vi "Variant_AdaptToType.vi"(7 "Default Type":variant, 10 "Variant":variant, 11 "Name (Default Type name)":string) -> (2 "Adapted Variant":variant)   [LabVIEW 2013, in "OpenVariant.lvlib"]
uses:
  OpenVariant.lvlib
  TypeDescriptor/TypeDescriptor_GetName.vi
  TypeDescriptor/TypeDescriptor_GetPString.vi
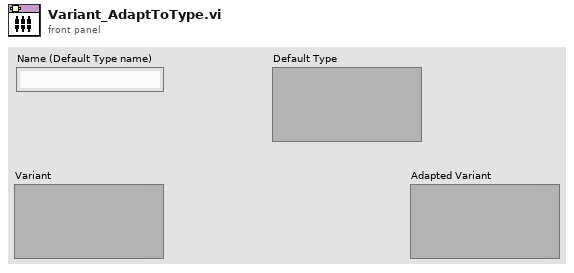
[diagram p1: front panel]
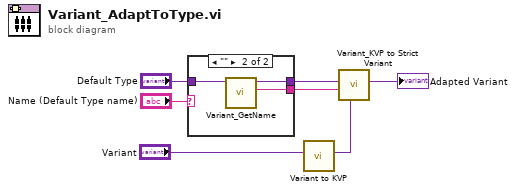
[diagram p0: block diagram]
diagram:
  n1 = case shown="\"\"" "Name (Default Type name)" {
    selector: "Name (Default Type name)" -> [w8 _]
    tunnel: "Default Type" -> [w9 w12]
    tunnel: [w9 w11] -> w4
    tunnel: [w8 w10] -> w3
    frame Default {
    }
    frame "" {
      n2 = call "Variant_GetName.vi"("Variant"=w12) -> ("Name"=w10:string, "Variant dup"=w11:variant)  [unwired: 8 in, 1 out]
    }
  }
  n3 = call "Variant to KVP.vi"("Variant"="Variant") -> ("KVP Dictionary"=w2:variant)  [unwired: 10 in]
  n4 = call "Variant_KVP to Strict Variant.vi"("KVP"=w2, "Default Value Name (empty: label)"=w3, "Default Value"=w4) -> ("Value"=→"Adapted Variant":variant)  [unwired: 5 in, 3 out]
